vi "Generate Discretes.vi"(9 "Connector m Bank n Discrete Stimulus":T1, 11 "Bank in":refnum<class "Bank.lvclass">) -> (3 "Bank out":refnum<class "Bank.lvclass">)   [LabVIEW 2019, in "LRUTS FPGA IP.lvlib" / "Bank.lvclass"]
uses:
  Bank.lvclass
  Discrete Generation Bank Control.ctl
  Bank Type.ctl
  Bank.lvclass/Bank.ctl
  <vilib>/rvi/eio/common/nirviEmuTemplateMethod_errors.vi
  <vilib>/eio/EIONode/EIONode.xnode
  <instrlib>/_niInstr/Basic Elements/v1/FPGA/niInstr Basic Elements v1 FPGA.lvlib
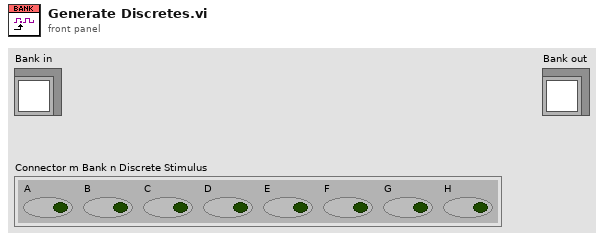
[diagram p1: front panel]
types:
  T1 = typedef "LRUTS FPGA IP.lvlib/Bank.lvclass/Discrete Generation Bank Control.ctl" = cluster{"A":bool, "B":bool, "C":bool, "D":bool, "E":bool, "F":bool, "G":bool, "H":bool}
  T2 = typedef "LRUTS FPGA IP.lvlib/Bank.lvclass/Bank Type.ctl" = enum16{"None", "Discrete Acquisition", "Discrete Generation", "PWM Acquisition", "PWM Generation"}
  T3 = typedef "LRUTS FPGA IP.lvlib/Bank.lvclass/FPGA IO Resources.ctl" = cluster{"DIO 0":refnum<k21>, "DIO 1":refnum<k21>, "DIO 2":refnum<k21>, "DIO 3":refnum<k21>, "DIO 4":refnum<k21>, "DIO 5":refnum<k21>, "DIO 6":refnum<k21>, "DIO 7":refnum<k21>}
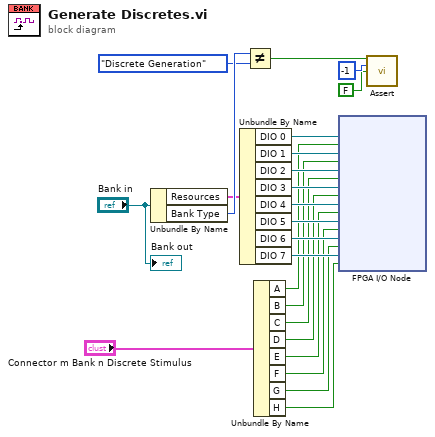
[diagram p0: block diagram]
diagram:
  n1 = Unbundle By Name("Bank in") -> ("Resources"=w18:T3, "Bank Type"=w23:T2)
  n2 = Unbundle By Name(w18) -> ("DIO 0"=w17:refnum<k21>, "DIO 1"=w16:refnum<k21>, "DIO 2"=w15:refnum<k21>, "DIO 3"=w14:refnum<k21>, "DIO 4"=w13:refnum<k21>, "DIO 5"=w12:refnum<k21>, "DIO 6"=w11:refnum<k21>, "DIO 7"=w10:refnum<k21>)
  n3 = Not Equal?(x=w23, y=Bank_Type."Discrete Generation") -> (x != y?=w21:bool)
  n4 = Unbundle By Name("Connector m Bank n Discrete Stimulus") -> ("A"=w8:bool, "B"=w7:bool, "C"=w6:bool, "D"=w5:bool, "E"=w4:bool, "F"=w3:bool, "G"=w2:bool, "H"=w1:bool)
  n5 = xnode "FPGA I/O Node"("I/O Item"=w8, "FPGA I/O In"=w17, "I/O Item"=w7, "FPGA I/O In"=w16, "I/O Item"=w6, "FPGA I/O In"=w15, "I/O Item"=w5, "FPGA I/O In"=w14, "I/O Item"=w4, "FPGA I/O In"=w13, "I/O Item"=w3, "FPGA I/O In"=w12, "I/O Item"=w2, "FPGA I/O In"=w11, "I/O Item"=w1, "FPGA I/O In"=w10) -> ()  [unwired: 8 out]
  n6 = call <instrlib>:"Assert.vi"("assert"=w21, "error code"=-1, "enable show error"=FALSE) -> ()  [unwired: 13 in]
  "Bank out" <- "Bank in"
